vi "DHE_DO_INTEGRATE.vi"(8 "error in (no error)":errorcluster) -> (0 "error IO":errorcluster, 2 "response":string)   [LabVIEW 2016]
uses:
  DBSHAND/private/vis/DatabaseHand_Element_Get(double).vi
  DBSHAND/private/vis/DatabaseHand_Element_Set(bool).vi
  DBSHAND/private/vis/DatabaseHand_Element_Set(double).vi
panel:
  in  "stopped":bool
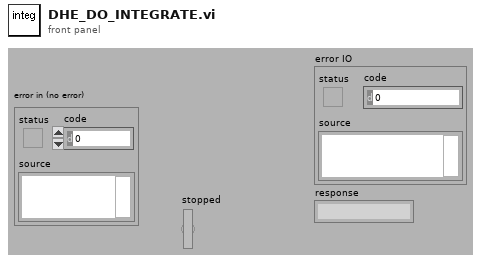
[diagram p1: front panel]
types:
  T1 = enum16{"Idle", "Exposing", "Paused", "AbortExp", "Reading", "AbortRead", "FinishedReading", "Resetting", "Reducing", "Initializing"}
  T2 = enum16{"get fd", "set fd", "add ", "set_readtime", "get all", "clean all", "get by fd"}
  T3 = typedef "DHE_Obs.ctl" = cluster{"observer":string, "obstype":string, "exptime":dbl, "coadds":i32, "fowler":i32, "nimages":i32, "display":bool, "autowrite":bool, "frames to write":cluster{"subs":bool, "reset":bool, "exposed":bool}, "frames to display":cluster{"subs":bool, "reset":bool, "exposed":bool}, "sur":i32}
  T4 = typedef "DatabaseHand_RefNum.ctl" = refnum<vi>
  T5 = typedef "DHE_Device.ctl" = cluster{"DevNo":i32, "fd":i32, "name":string, "FPA":string, "modifiers":string, "binpatt":string, "readtime":dbl, "readmode":string, "type":string, "params":string}
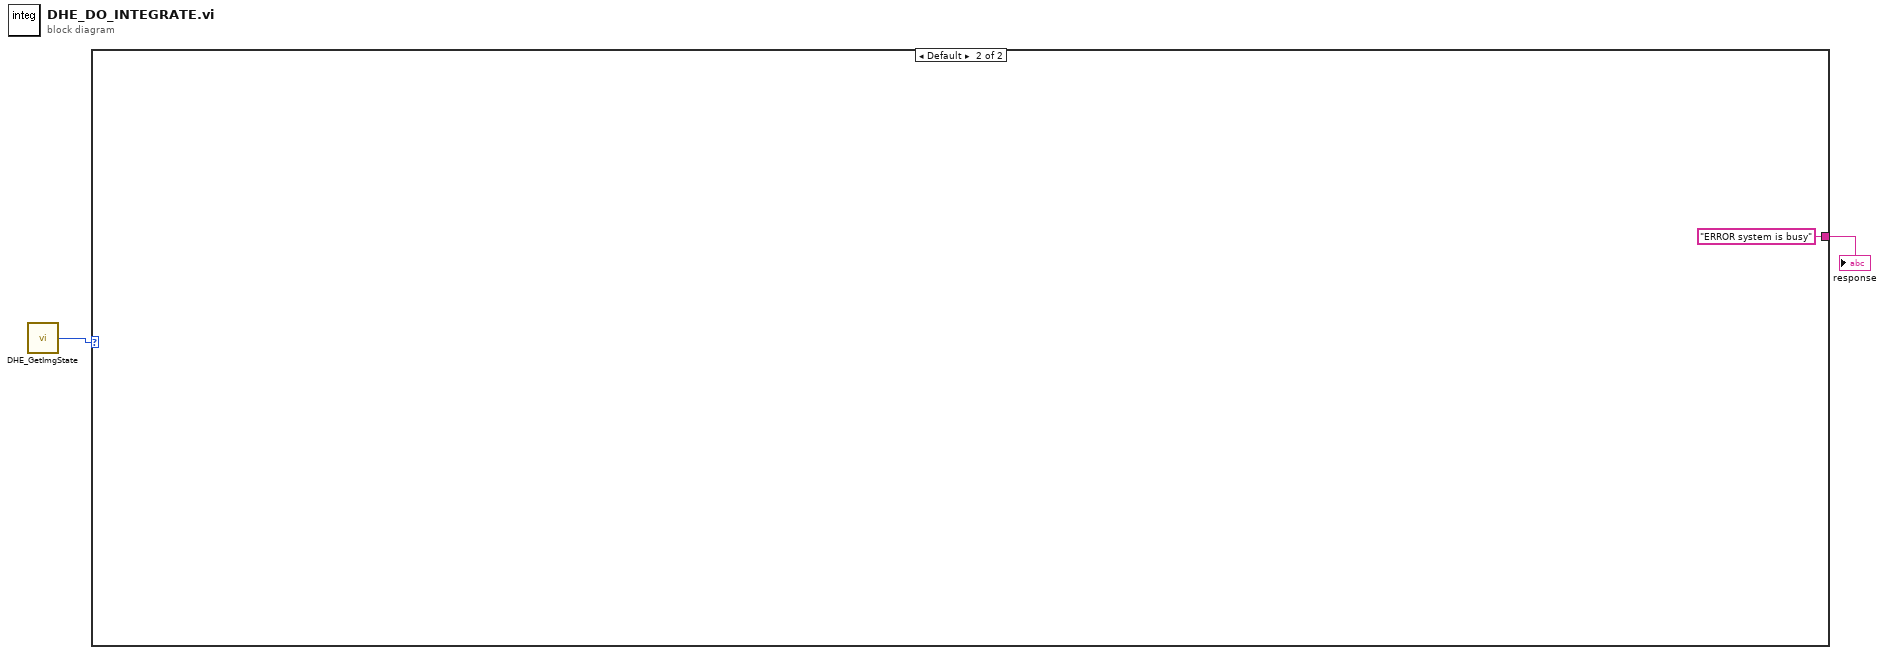
[diagram p0: block diagram]
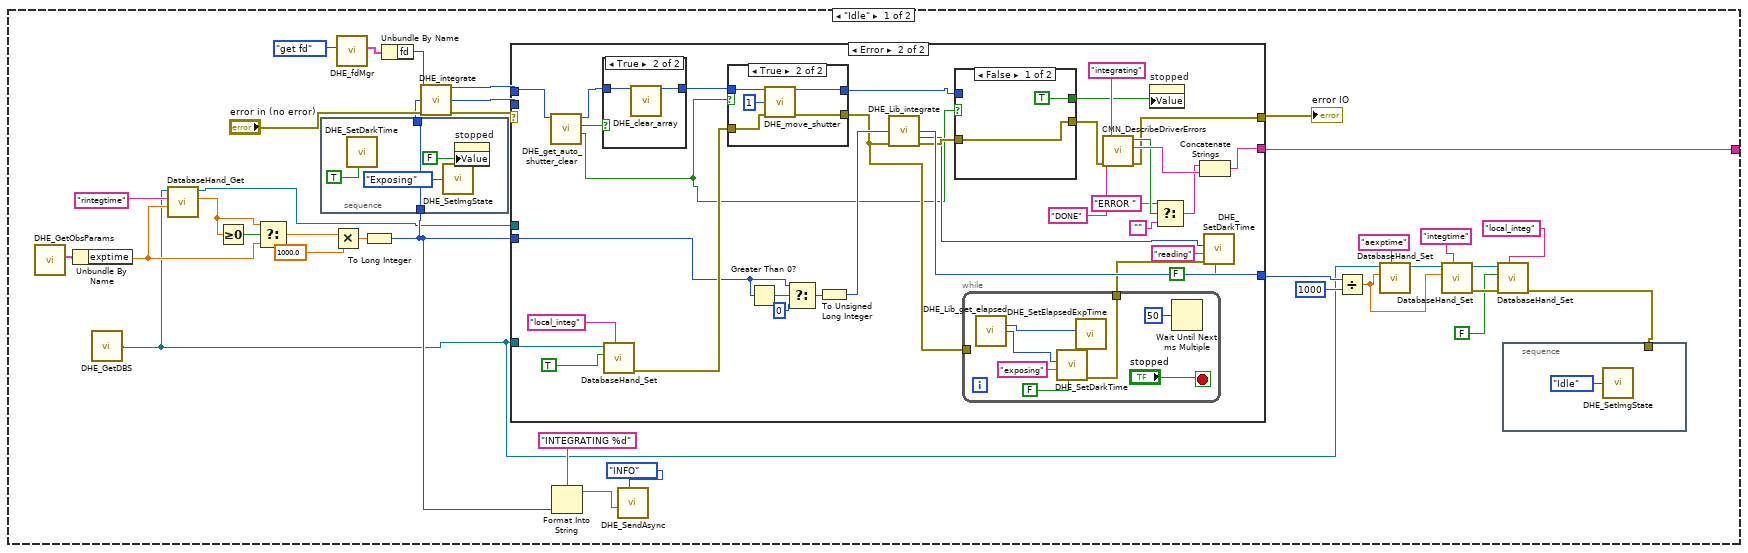
[diagram p2: hidden frame]
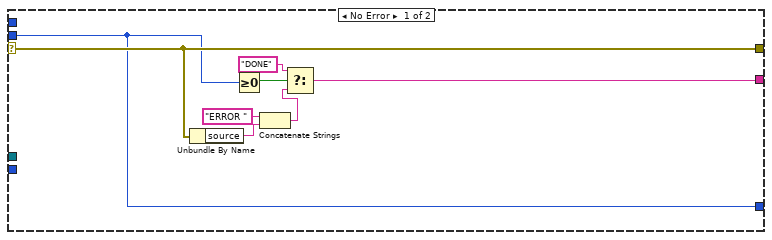
[diagram p3: hidden frame]
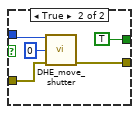
[diagram p5: hidden frame]
diagram:
  n1 = call "DHE_GetImgState.vi"() -> ("DHE_ImgState"=w1:T1)  [unwired: 9 out]
  n2 = case shown="Default" w1 {
    tunnel: [w37 "ERROR system is busy"] -> w2
    frame "Idle" {
      n3 = call "DHE_GetObsParams.vi"() -> ("DHE_OBS"=w13:T3)  [unwired: 11 out]
      n4 = Unbundle By Name(w13) -> ("exptime"=w8:dbl)
      n5 = call "DHE_GetDBS.vi"() -> ("DHE_DBSRef"=w4:T4)  [unwired: 9 out]
      n6 = call-poly "DatabaseHand_Get.vi"("default value"=w8, "name"="rintegtime", "Database RefNum in"=w4) -> ("value"=w9:dbl, "Database RefNum out"=w3:T4)  [unwired: 2 in, 5 out]
      n7 = Greater Or Equal To 0?(x=w9) -> (x >= 0?=w10:bool)
      n8 = Select(t=w9, s=w10, f=w8) -> (s? t:f=w7:dbl)
      n9 = Multiply(x=w7, y=1000.0) -> (x*y=w11:dbl)
      n10 = call "DHE_fdMgr.vi"("action"=T2."get fd") -> ("Device"=w27:T5)  [unwired: 4 in, 6 out]
      n11 = To Long Integer(number=w11) -> (32bit integer=w34:i32)
      n12 = stacked-sequence {
        tunnel: w34 -> [w40]
        tunnel: [w40] -> w5
        frame #0 {
          n13 = call "DHE_SetDarkTime.vi"("flush?"=TRUE) -> ()  [unwired: 3 in, 8 out]
          n14 = call "DHE_SetImgState.vi"("DHE_ImgState"=T1."Exposing") -> ()  [unwired: 9 out]
          n15 = property on="stopped" class="Bool (strict)"("Value"=FALSE ("stopped")) -> ()  [unwired: 2 in, 2 out]
        }
      }
      n16 = Unbundle By Name(w27) -> ("fd"=w26:i32)
      n17 = call "DHE_integrate.vi"("fd"=w26, "msecs"=w5, "error in (no error)"="error in (no error)") -> ("fd out"=w31:i32, "return value"=w29:i32, "error out"=w32:errorcluster)  [unwired: 10 out]
      n18 = case shown="Error" w32 {
        selector: w32 -> [w48 _]
        tunnel: w31 -> [_ w55]
        tunnel: [w48 w61] -> w30
        tunnel: w29 -> [w43 _]
        tunnel: [w44 w75] -> w37
        tunnel: [w43 w72] -> w23
        tunnel: w4 -> [_ w71]
        tunnel: w34 -> [_ w67]
        tunnel: w3 -> [_ _]
        frame No Error {
          n19 = Unbundle By Name(w48) -> ("source"=w47:string)
          n20 = Greater Or Equal To 0?(x=w43) -> (x >= 0?=w50:bool)
          n21 = Concatenate Strings("ERROR " ("string"), w47) -> (w45:string)
          n22 = Select(t="DONE", s=w50, f=w45) -> (s? t:f=w44:string)
        }
        frame Error {
          n23 = call "DHE_get_auto_shutter_clear.vi"("fd"=w55) -> ("autoshutter"=w54:bool, "autoclear"=w52:bool, "fd out"=w53:i32)  [unwired: 1 in, 7 out]
          n24 = case shown="True" w52 {
            tunnel: w53 -> [w84 w86]
            tunnel: [w84 w85] -> w51
            frame False {
            }
            frame True {
              n25 = call "DHE_clear_array.vi"("fd"=w86) -> ("fd out"=w85:i32)  [unwired: 1 in, 13 out]
            }
          }
          n26 = call-poly "DatabaseHand_Set.vi"("name"="local_integ", "value"=TRUE, "Database RefNum in"=w71) -> ("error out"=w68:errorcluster)  [unwired: 5 in, 3 out]
          n27 = case shown="True" w54 {
            tunnel: w51 -> [w102 w107]
            tunnel: [w102 w105] -> w83
            tunnel: [w101 w104] -> w63
            tunnel: w68 -> [w101 w103]
            frame False {
            }
            frame True {
              n28 = call "DHE_move_shutter.vi"("fd"=w107, "flag"=i16 1, "error in (no error)"=w103) -> ("fd out"=w105:i32, "error out"=w104:errorcluster)  [unwired: 11 out]
            }
          }
          n29 = Greater Than 0?(x=w67) -> (x > 0?=w74:bool)
          n30 = Select(t=w67, s=w74, f=0) -> (s? t:f=w66:i32)
          n31 = To Unsigned Long Integer(number=w66) -> (unsigned 32bit integer=w65:u32)
          n32 = call "DHE_Lib_integrate.vi"("msecs"=w65, "error in (no error)"=w63) -> ("return value"=w72:i32, "dark time"=w57:i32, "error out"=w62:errorcluster)  [unwired: 11 out]
          n33 = case shown="False" w54 {
            tunnel: w83 -> [_ w100]
            tunnel: [w95 w98] -> w64
            tunnel: w62 -> [w95 w97]
            tunnel: [TRUE ("stopped") TRUE ("stopped")] -> w60
            frame False {
            }
            frame True {
              n34 = call "DHE_move_shutter.vi"("fd"=w100, "flag"=i16 0, "error in (no error)"=w97) -> ("error out"=w98:errorcluster)  [unwired: 12 out]
            }
          }
          n35 = while {
            tunnel: w63 -> [_]
            tunnel: [w88] -> w59
            stop <- "stopped" stop-if-true
            n36 = call "DHE_Lib_get_elapsed.vi"() -> ("elapsed"=w90:i32, "darktime"=w87:i32)  [unwired: 1 in, 13 out]
            n37 = call "DHE_SetDarkTime.vi"("flush?"=FALSE, "detstat"="exposing", "darktime"=w87) -> ("error out"=w88:errorcluster)  [unwired: 1 in, 7 out]
            n38 = call "DHE_SetElapsedExpTime.vi"("ElapsedExpTime"=w90) -> ()  [unwired: 11 out]
            n39 = Wait Until Next ms Multiple(millisecond multiple=u32 50) -> ()  [unwired: 1 out]
          }
          n40 = call "CMN_DescribeDriverErrors.vi"("message"="integrating", "OK message"="DONE", "error in (no error)"=w64) -> ("error?"=w79:bool, "astroerrors"=w80:string, "error out"=w61:errorcluster)  [unwired: 1 in, 4 out]
          n41 = property on="stopped" class="Bool (strict)"("Value"=w60) -> ()  [unwired: 2 in, 2 out]
          n42 = Select(t="ERROR ", s=w79, f="") -> (s? t:f=w76:string)
          n43 = Concatenate Strings(w76, w80) -> (w75:string)
          n44 = call "DHE_SetDarkTime.vi"("flush?"=FALSE, "error in (no error)"=w59, "detstat"="reading", "darktime"=w57) -> ()  [unwired: 8 out]
        }
      }
      "error IO" <- w30
      n45 = Format Into String(format string="INTEGRATING %d", w34) -> (resulting string=w33:string)  [unwired: 2 in, 1 out]
      n46 = call "DHE_SendAsync.vi"("type"=enum16{"ERROR", "WARNING", "INFO", "CHANGED"}."INFO", "Message"=w33) -> ()  [unwired: 2 in, 8 out]
      n47 = Divide(x=w23, y=1000) -> (x/y=w20:dbl)
      n48 = call-poly "DatabaseHand_Set.vi"("name"="aexptime", "value"=w20, "Database RefNum in"=w4) -> ("Database RefNum out"=w21:T4)  [unwired: 5 in, 3 out]
      n49 = call-poly "DatabaseHand_Set.vi"("name"="integtime", "value"=w20, "Database RefNum in"=w21) -> ("error out"=w19:errorcluster, "Database RefNum out"=w18:T4)  [unwired: 5 in, 2 out]
      n50 = call-poly "DatabaseHand_Set.vi"("name"="local_integ", "error in (no error)"=w19, "value"=FALSE, "Database RefNum in"=w18) -> ("error out"=w6:errorcluster)  [unwired: 4 in, 3 out]
      n51 = stacked-sequence {
        tunnel: w6 -> [_]
        frame #0 {
          n52 = call "DHE_SetImgState.vi"("DHE_ImgState"=T1."Idle") -> ()  [unwired: 9 out]
        }
      }
    }
    frame Default {
    }
  }
  "response" <- w2
